vi "From Variant.vi"(0 "TTLDevice in":refnum<class "TTLControlledDevice.lvclass">, 7 "Variant":variant, 9 "Prefix":string, 11 "error in (no error)":errorcluster) -> (4 "TTLDevice out":refnum<class "TTLControlledDevice.lvclass">, 15 "error out":errorcluster)   [LabVIEW 2020, in "TTLControlledDevice.lvclass"]
uses:
  TTLControlledDevice.lvclass
  TTLControlledDevice.lvclass/TTLControlledDevice.ctl
  epl-vi-lib/Koop/KObject Class/KObject.lvclass
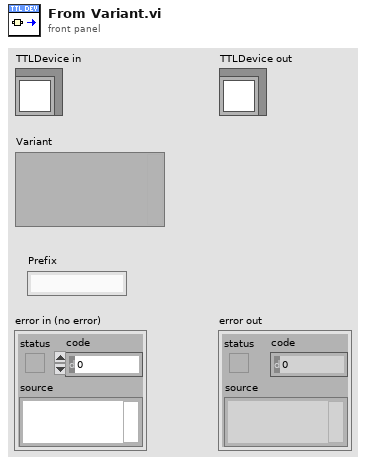
[diagram p1: front panel]
types:
  T1 = typedef "TTLControlledDevice.lvclass/Serialized.ctl" = cluster{"Name":string, "Line":string}
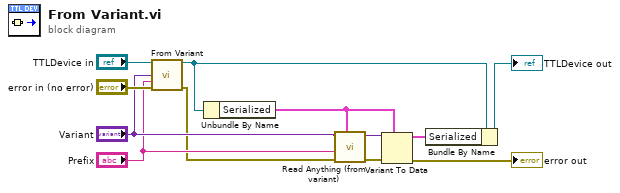
[diagram p0: block diagram]
diagram:
  n1 = call-parent "From Variant.vi"("KObject in"="TTLDevice in", "Variant"="Variant", "Prefix"="Prefix", "error in (no error)"="error in (no error)") -> ("KObject out"=w7:refnum<class "TTLControlledDevice.lvclass">, "error out"=w4:errorcluster)  [unwired: 10 in]
  n2 = Unbundle By Name(w7) -> ("Serialized"=w8:T1)
  n3 = call "Read Anything (from variant).vi"("Type of Anything"=w8, "Error In"=w4, "Prefix"="Prefix", "Variant Database"="Variant") -> ("Error Out"=w9:errorcluster, "Anything"=w10:variant)  [unwired: 5 in, 1 out]
  n4 = Variant To Data(error in=w9, type=w8, Variant=w10) -> (data=w1:T1, error out=→"error out":errorcluster)
  n5 = Bundle By Name(cluster=w7, "Serialized"=w1) -> (→"TTLDevice out":refnum<class "TTLControlledDevice.lvclass">)
